vi "RT RFIDs.vi"(8 "error in (no error)":errorcluster, 10 "info":cluster{"File path":T3, "Cfg ":T4} {"Cfg"."Offset_rueda WS 2" format="%.27g"; "Cfg"."Offset_rueda WS 1" format="%.27g"; "Cfg"."Frecuencia de muestreo y módulo CRIO" items=["51.200 kS/s (NI 9234)"=1, "25.600 kS/s (NI 9234)"=2, "17.067 kS/s (NI 9234)"=3, "12.800 kS/s (NI 9234)"=4, "10.240 kS/s (NI 9234)"=5, "8.533 kS/s (NI 9234)"=6, "7.314 kS/s (NI 9234)"=7, "6.400 kS/s (NI 9234)"=8, "5.689 kS/s (NI 9234)"=9, "5.120 kS/s (NI 9234)"=10, "4.654 kS/s (NI 9234)"=11, "4.267 kS/s (NI 9234)"=12, "3.938 kS/s (NI 9234)"=13, "3.657 kS/s (NI 9234)"=14, "3.413 kS/s (NI 9234)"=15, "3.200 kS/s (NI 9234)"=16, "3.012 kS/s (NI 9234)"=17, "2.845 kS/s (NI 9234)"=18, "2.695 kS/s (NI 9234)"=19, "2.560 kS/s (NI 9234)"=20, "2.438 kS/s (NI 9234)"=21, "2.328 kS/s (NI 9234)"=22, "2.226 kS/s (NI 9234)"=23, "2.133 kS/s (NI 9234)"=24, "2.048 kS/s (NI 9234)"=25, "1.969 kS/s (NI 9234)"=26, "1.896 kS/s (NI 9234)"=27, "1.829 kS/s (NI 9234)"=28, "1.765 kS/s (NI 9234)"=29, "1.707 kS/s (NI 9234)"=30, "1.652 kS/s (NI 9234)"=31]}, 11 "Message Queues in":T6) -> (0 "error out":errorcluster)   [LabVIEW 2015]
uses:
  support/Message Queue/All Message Queues.ctl
  support/Message Queue/Message Cluster.ctl
  controls/File paths.ctl
  controls/Cfg_parameters.ctl
  <vilib>/LabVIEW Targets/FPGA/cRIO/shared/nicrio_ModuleControls/nicrio_cRIO-9234_DataRatesRing2.ctl
  controls/RFID State.ctl
  controls/Tags.ctl
  <vilib>/Utility/file.llb/Write Delimited Spreadsheet (string).vi
  support/Message Queue/Enqueue Message (Single).vi
  <vilib>/Utility/error.llb/Error Cluster From Error Code.vi
  <vilib>/ErrorRing/Error Ring.xnode
  support/Message Queue/Message Queue.lvlib
panel:
  in  "TAGs":T1
  in  "RFID State":T2
  out "RFID_LR6_Error":errorcluster
  out "RFID_Error":errorcluster
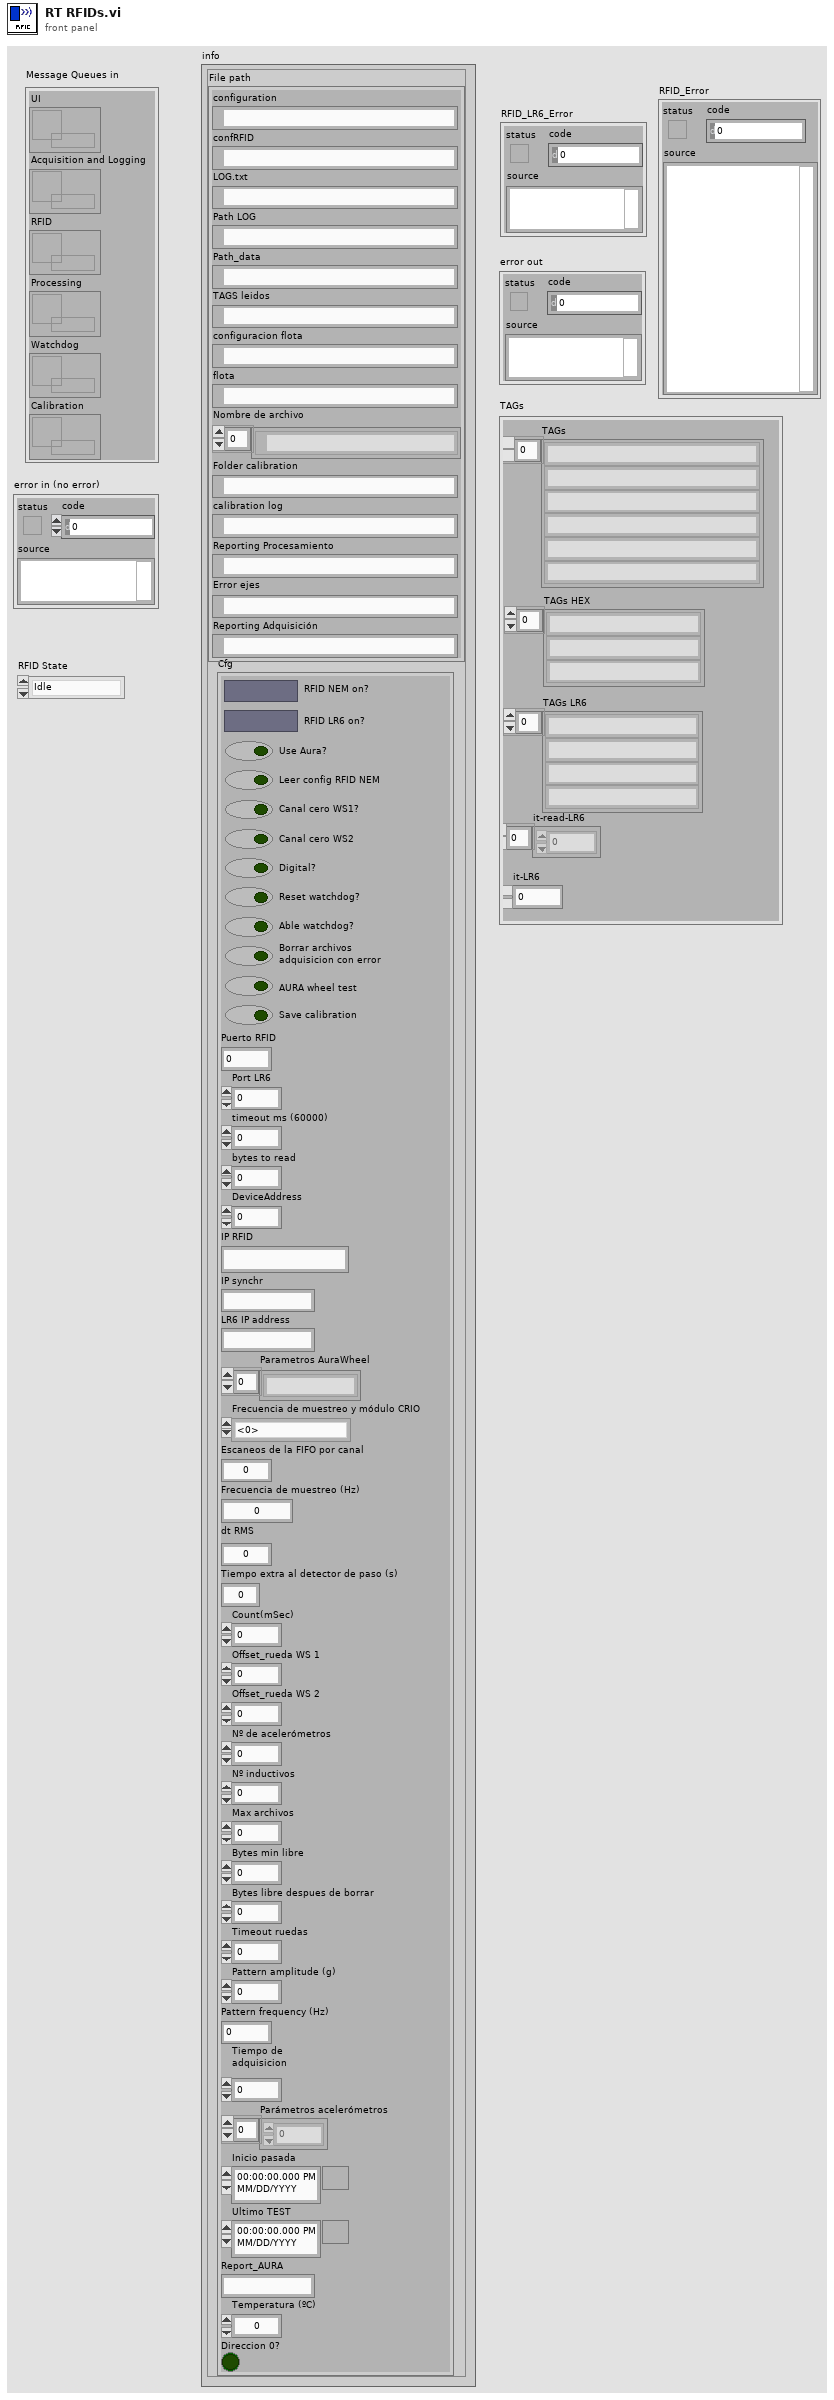
[diagram p1: front panel]
types:
  T1 = typedef "Tags.ctl" = cluster{"TAGs":string[], "TAGs HEX":string[], "TAGs LR6":string[], "it-read-LR6":i32[], "it-LR6":i32}
  T2 = typedef "RFID State.ctl" = enum16{"Idle", "Acquiring"}
  T3 = typedef "File paths.ctl" = cluster{"configuration":path, "confRFID":path, "LOG.txt":path, "Path LOG":path, "Path_data":path, "TAGS leidos":path, "configuracion flota":path, "flota":path, "Nombre de archivo":path[], "Folder calibration":path, "calibration log":path, "Reporting Procesamiento":path, "Error ejes":path, "Reporting Adquisición":path}
  T4 = typedef "Cfg_parameters.ctl" = cluster{"RFID NEM on?":bool, "RFID LR6 on?":bool, "Use Aura?":bool, "Leer config RFID NEM":bool, "Canal cero WS1?":bool, "Canal cero WS2 ":bool, "Digital?":bool, "Reset watchdog?":bool, "Able watchdog?":bool, "Borrar archivos\nadquisicion con error":bool, "AURA wheel test":bool, "Save calibration":bool, "Puerto RFID":u16, "Port LR6":u16, "timeout ms (60000)":i32, "bytes to read":i32, "DeviceAddress":u8, "IP RFID":string, "IP synchr":string, "LR6 IP address":string, "Parametros AuraWheel":string[], "Frecuencia de muestreo y módulo CRIO":T5, "Escaneos de la FIFO por canal":u32, "Frecuencia de muestreo (Hz)":dbl, "dt RMS":dbl, "Tiempo extra al detector de paso (s)":dbl, "Count(mSec)":u32, "Offset_rueda WS 1":fxp<+/-,24,-4>, "Offset_rueda WS 2":fxp<+/-,24,-4>, "Nº de acelerómetros":i32, "Nº inductivos":i32, "Max archivos":u32, "Bytes min libre":u32, "Bytes libre despues de borrar":u32, "Timeout ruedas":dbl, "Pattern amplitude (g)":dbl, "Pattern frequency (Hz)":dbl, "Tiempo de adquisicion\n":dbl, "Parámetros acelerómetros":dbl[], "Inicio pasada":timestamp, "Ultimo TEST":timestamp, "Report_AURA":string, "Temperatura (ºC)":dbl, "Direccion 0?":bool}
  T5 = typedef "nicrio_cRIO-9234_DataRatesRing2.ctl" = u8
  T6 = typedef "Message Queue.lvlib/All Message Queues.ctl" = cluster{"UI":refnum<queue>, "Acquisition and Logging":refnum<queue>, "RFID":refnum<queue>, "Processing":refnum<queue>, "Watchdog":refnum<queue>, "Calibration":refnum<queue>}
  T7 = enum16{"Standard", "Buffered", "CRLF", "Immediate"}
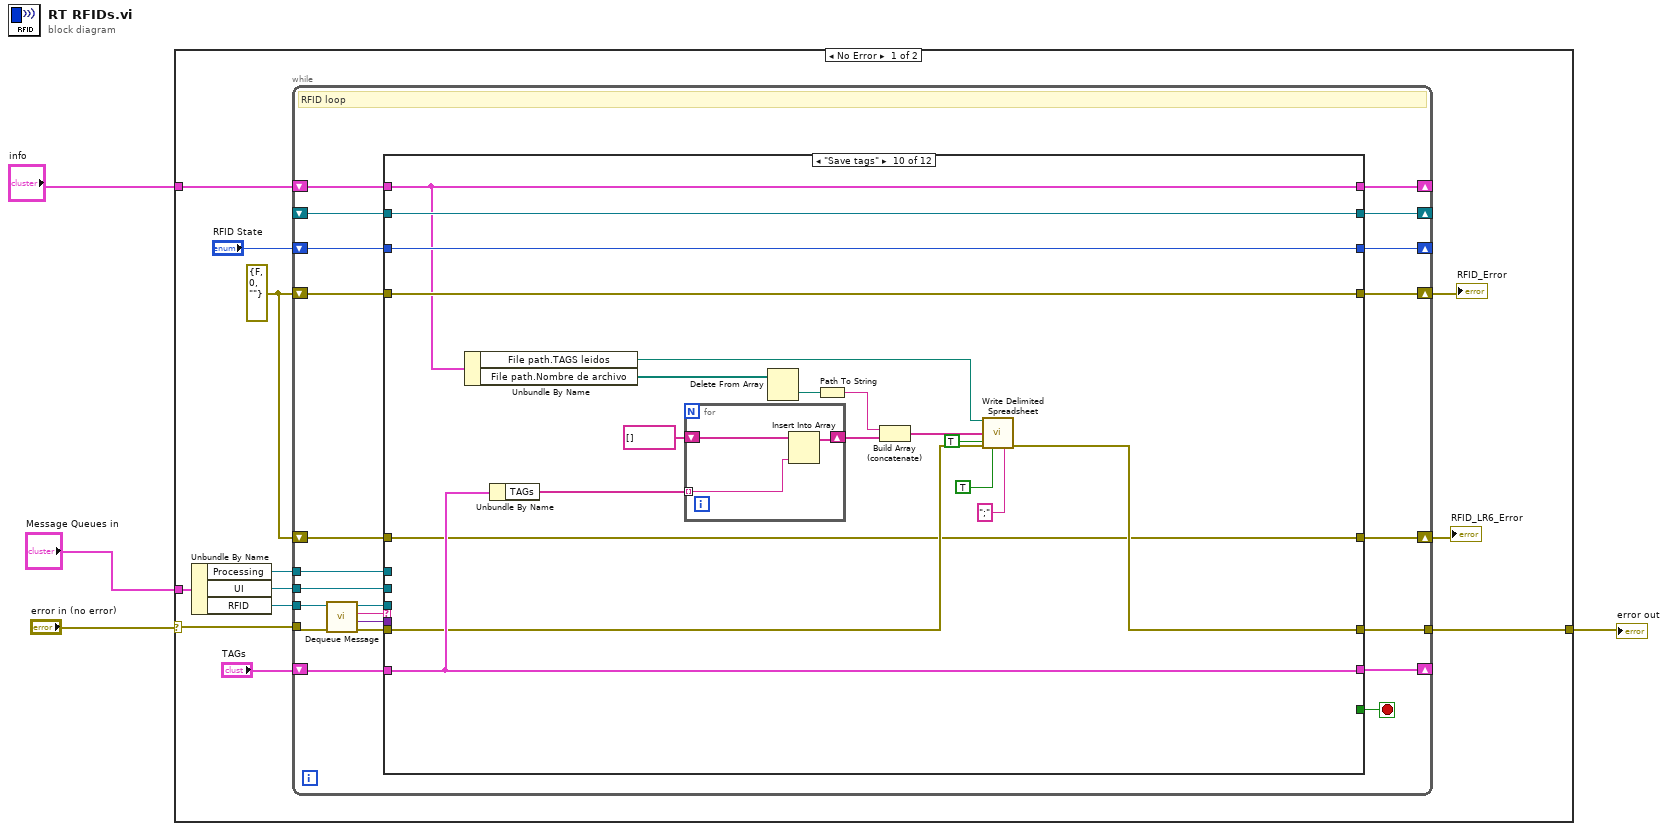
[diagram p0: block diagram]
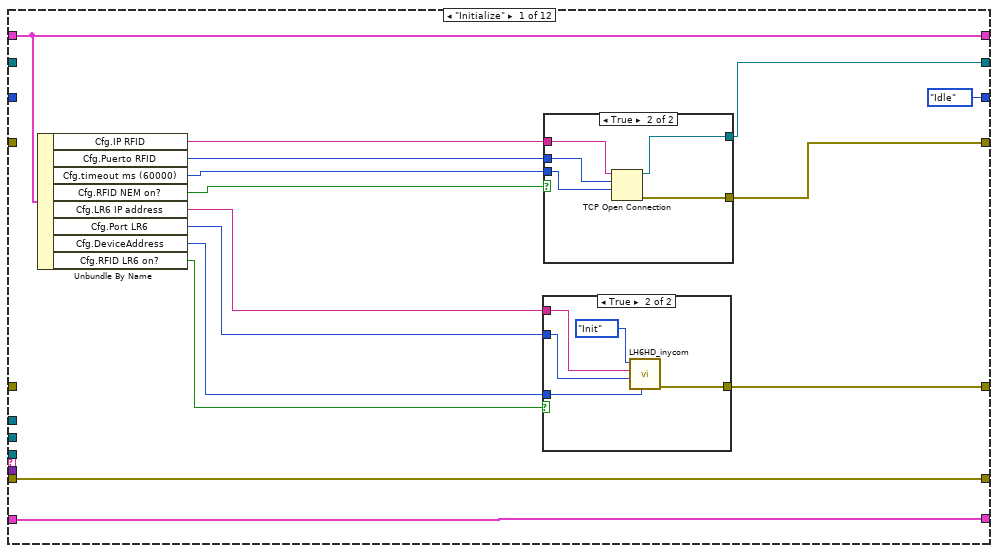
[diagram p2: hidden frame]
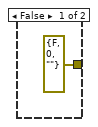
[diagram p3: hidden frame]
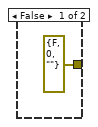
[diagram p4: hidden frame]
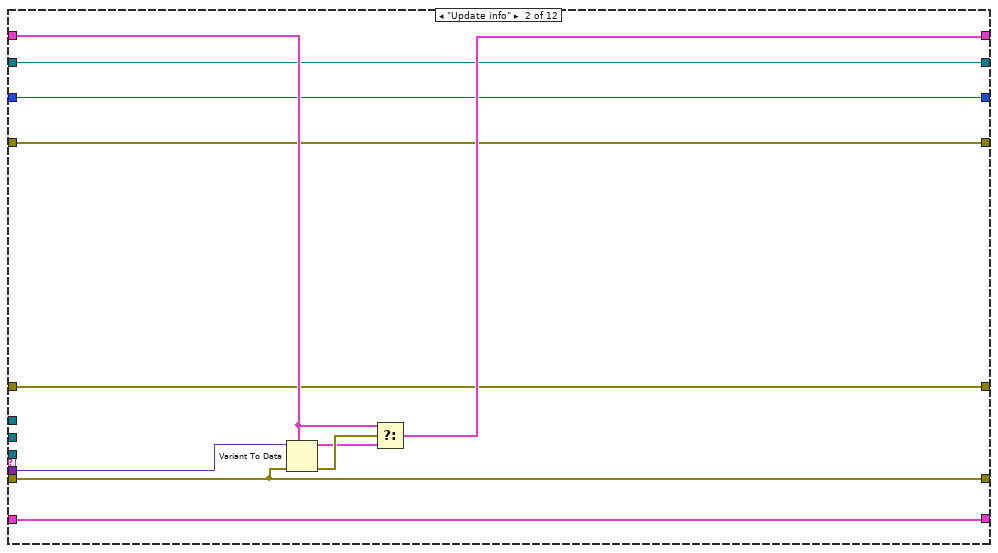
[diagram p5: hidden frame]
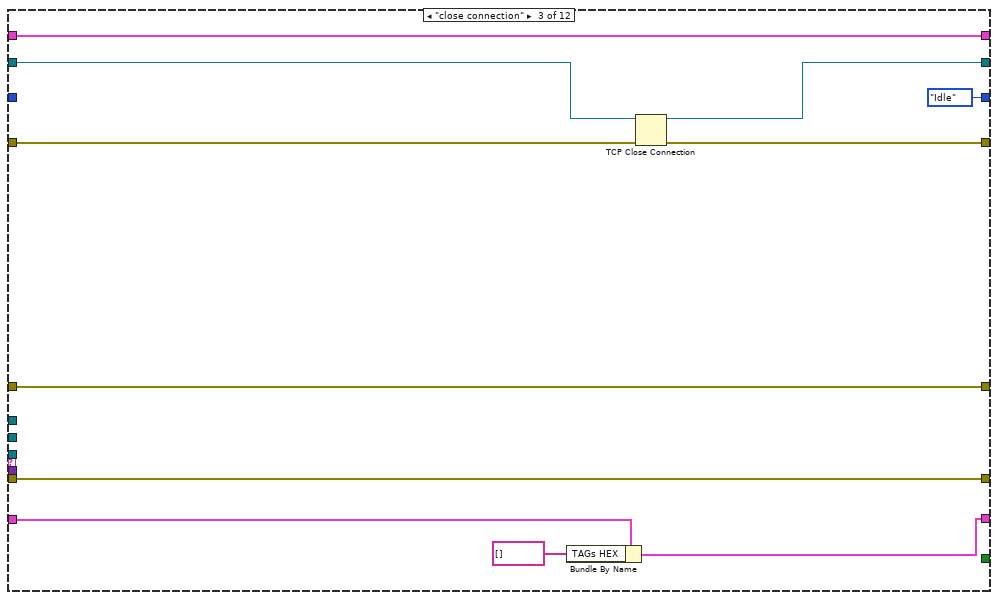
[diagram p6: hidden frame]
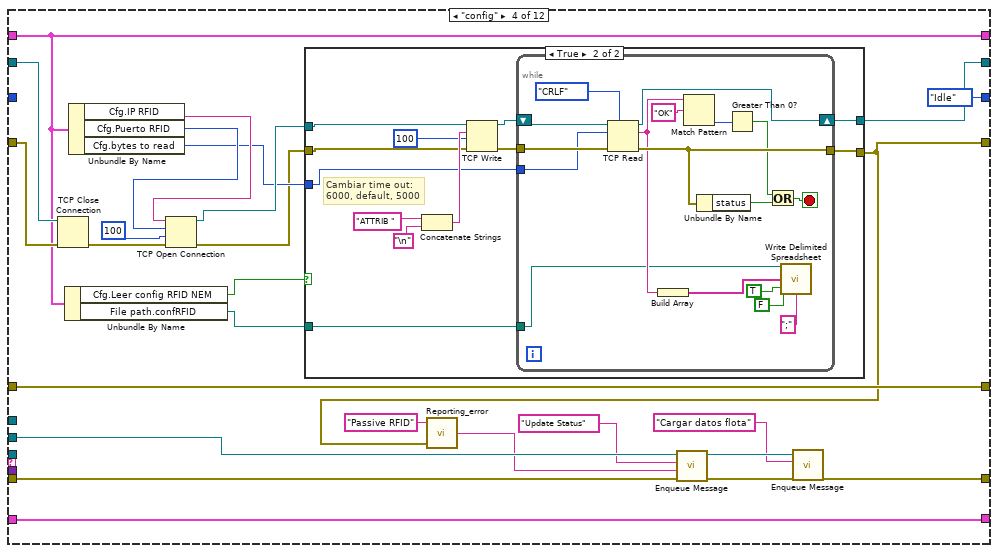
[diagram p7: hidden frame]
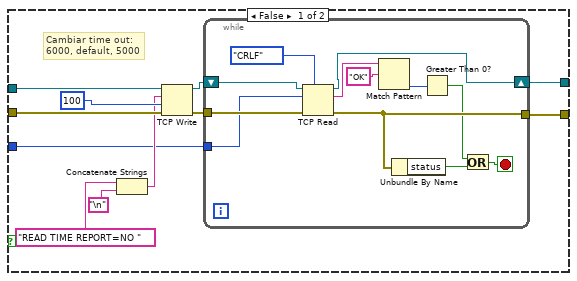
[diagram p8: hidden frame]
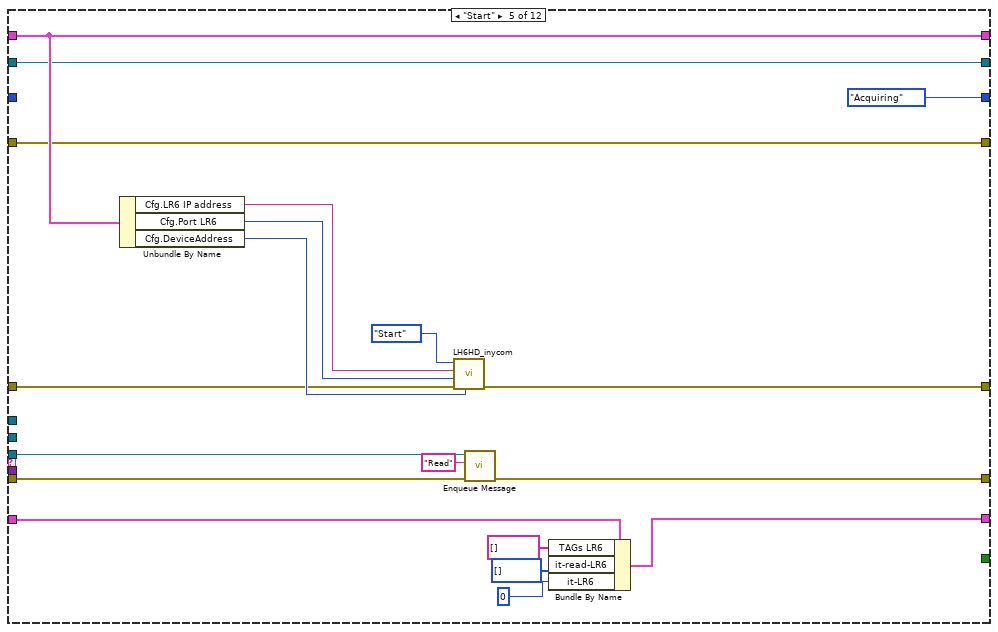
[diagram p9: hidden frame]
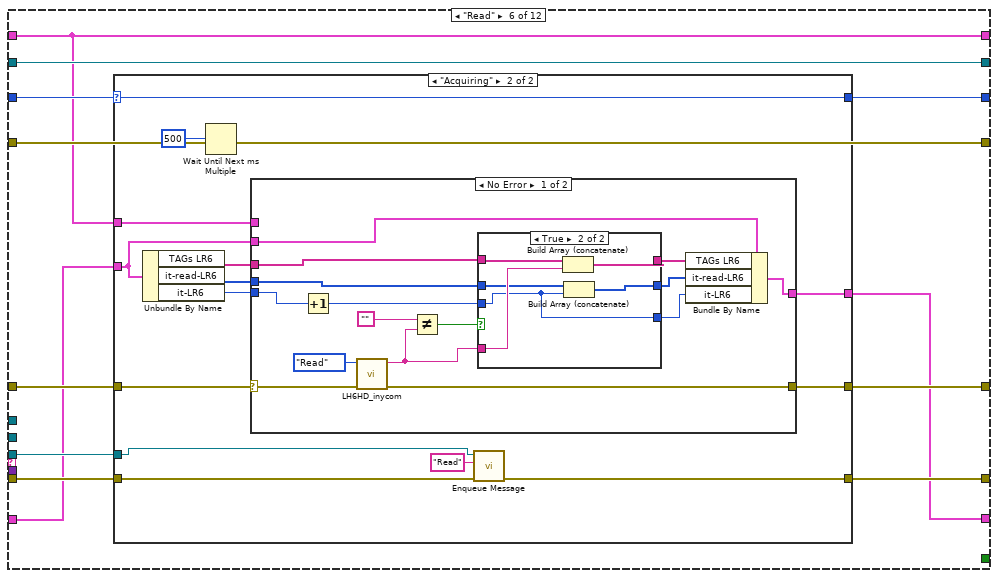
[diagram p10: hidden frame]
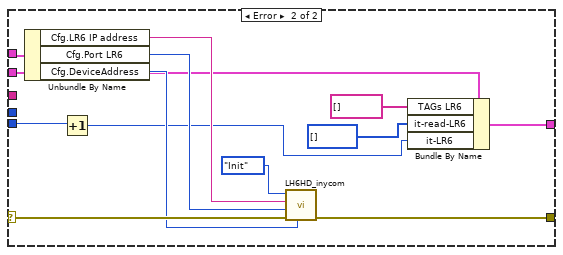
[diagram p13: hidden frame]
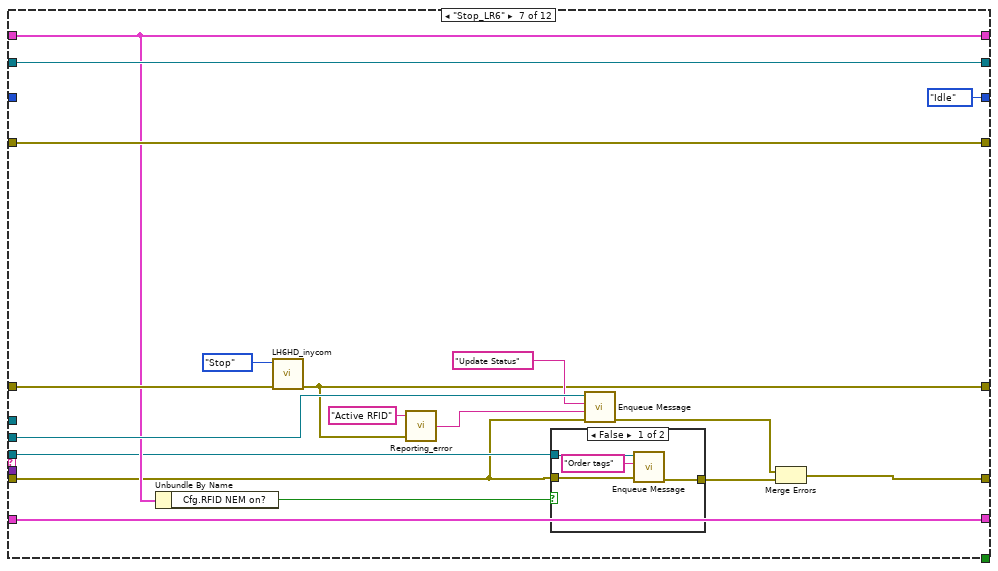
[diagram p14: hidden frame]
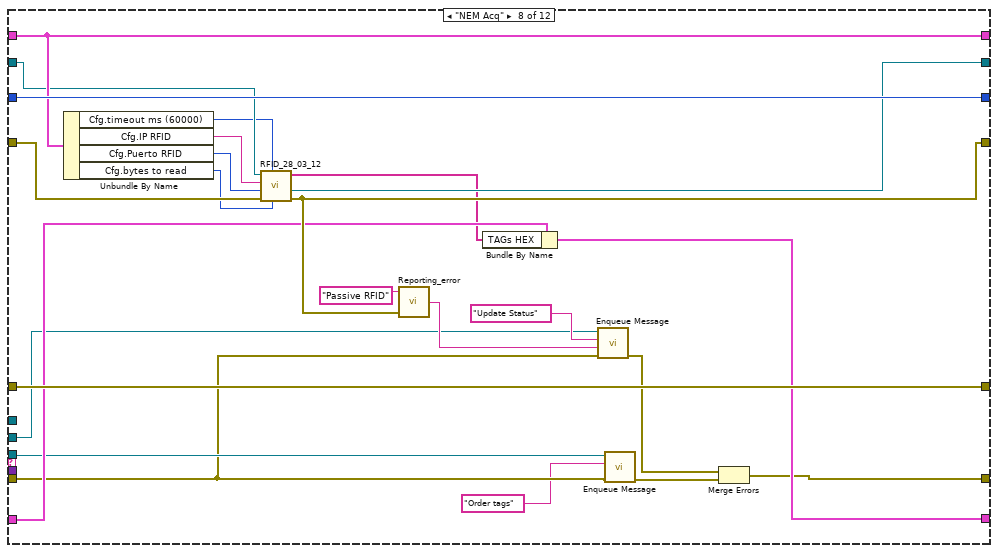
[diagram p16: hidden frame]
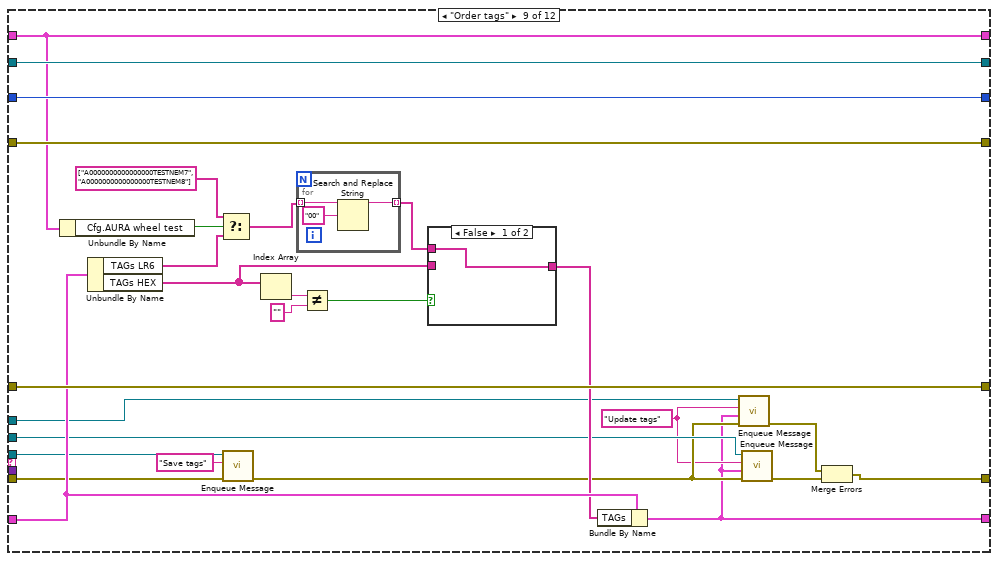
[diagram p17: hidden frame]
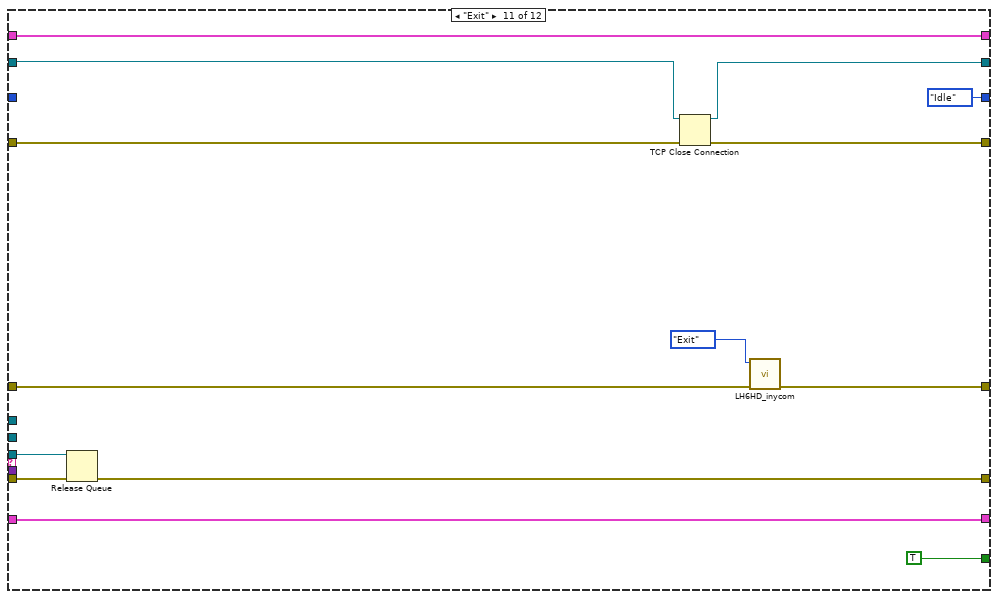
[diagram p19: hidden frame]
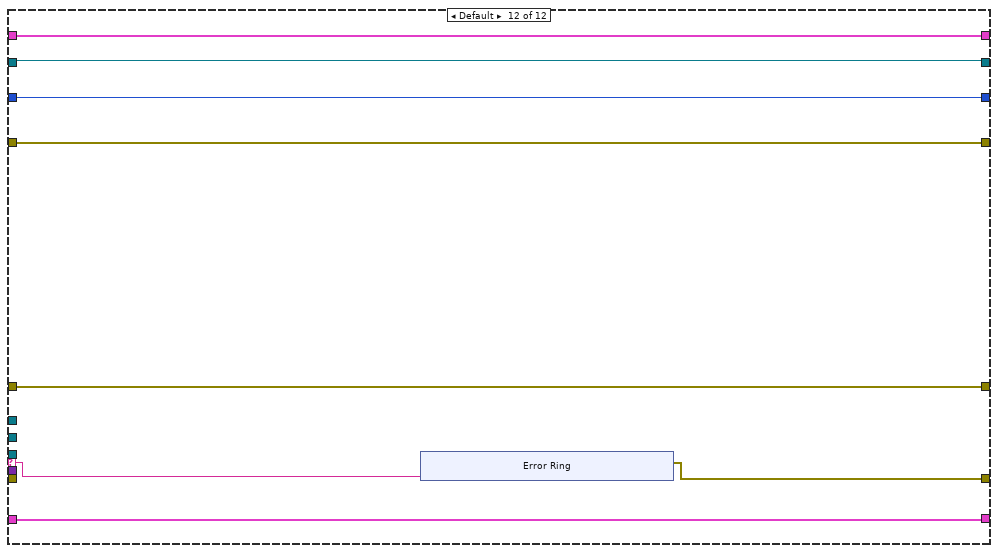
[diagram p20: hidden frame]
diagram:
  n1 = case shown="No Error" "error in (no error)" {
    selector: "error in (no error)" -> [w15 w382]
    tunnel: "Message Queues in" -> [w16 _]
    tunnel: "info" -> [w12 _]
    tunnel: [w11 w382] -> w1
    frame No Error {
      w8 = errorcluster {"status"=FALSE, "code"=0, "source"=""} ("error out")
      n2 = Unbundle By Name(w16) -> ("Processing"=w5:refnum<queue>, "UI"=w13:refnum<queue>, "RFID"=w14:refnum<queue>)
      n3 = while {
        tunnel: w15 -> [w38]
        tunnel: w14 -> [w37]
        tunnel: w13 -> [w35]
        shift-right: [w31] -> _
        shift-left: w12 -> [w32]
        tunnel: [w29] -> w11
        shift-right: [w28] -> _
        shift-left: _ -> [w27]
        shift-right: [w25] -> w9
        shift-left: w8 -> [w24]
        shift-right: [w26] -> w10
        shift-left: w8 -> [w23]
        shift-right: [w21] -> _
        shift-left: "RFID State" -> [w22]
        shift-right: [w19] -> _
        shift-left: "TAGs" -> [w20]
        tunnel: w5 -> [w17]
        stop <- w30 stop-if-true
        # "RFID loop"
        n4 = call "Dequeue Message.vi"("error in (no error)"=w38, "Message Queue"=w37) -> ("error out"=w34:errorcluster, "Message Data"=w18:variant, "Message"=w33:string, "dup Message Queue"=w36:refnum<queue>)  [unwired: 6 in]
        n5 = case shown="\"Save tags\"" w33 {
          selector: w33 -> [_ _ _ _ _ _ _ _ _ _ _ w372]
          tunnel: w36 -> [_ _ _ _ w174 w188 w257 w280 w305 _ w364 _]
          tunnel: w35 -> [_ _ _ w94 _ _ w262 w281 w308 _ _ _]
          tunnel: w34 -> [w53 w73 w83 w91 w176 w190 w256 w276 w307 w333 w365 _]
          tunnel: [w53 w73 w83 w90 w175 w189 w253 w279 w299 w332 w363 w373] -> w29
          tunnel: w32 -> [w52 w70 w87 w102 w180 w187 w258 w295 w321 w336 w366 w374]
          tunnel: [w52 w71 w87 w102 w180 w187 w258 w295 w321 w336 w366 w374] -> w31
          tunnel: [_ _ _ _ _ _ _ _ _ _ TRUE _] -> w30
          tunnel: [w47 w67 w86 w98 w178 w193 w267 w293 w323 w347 w361 w370] -> w25
          tunnel: [w46 w68 w85 w103 w177 w194 w268 w292 w325 w349 w360 w371] -> w28
          tunnel: w27 -> [_ w68 w84 w110 w177 w194 w268 w291 w325 w349 w359 w371]
          tunnel: [w41 w66 w81 w113 w181 w191 w260 w297 w322 w331 w357 w369] -> w26
          tunnel: w24 -> [_ w67 w82 w105 w178 w193 w267 w294 w323 w347 w356 w370]
          tunnel: w23 -> [_ w66 w81 w113 w179 w192 w265 w297 w322 w331 w355 w369]
          tunnel: w22 -> [_ w69 _ _ _ w196 _ w298 w324 w348 _ w368]
          tunnel: [RFID_State."Idle" ("RFID State") w69 RFID_State."Idle" ("RFID State") RFID_State."Idle" ("RFID State") RFID_State."Acquiring" ("RFID State") w195 RFID_State."Idle" ("RFID State") w298 w324 w348 RFID_State."Idle" ("RFID State") w368] -> w21
          tunnel: w20 -> [w39 w72 w79 w88 w172 w186 w263 w284 w311 w338 w353 w367]
          tunnel: [w39 w72 w78 w88 w171 w185 w263 w282 w302 w338 w353 w367] -> w19
          tunnel: w18 -> [_ w74 _ _ _ _ _ _ _ _ _ _]
          tunnel: w17 -> [_ _ _ _ _ _ _ _ w309 _ _ _]
          frame "Initialize" {
            n6 = Unbundle By Name(w52) -> ("Cfg.IP RFID"=w51:string, "Cfg.Puerto RFID"=w49:u16, "Cfg.timeout ms (60000)"=w48:i32, "Cfg.RFID NEM on?"=w50:bool, "Cfg.LR6 IP address"=w44:string, "Cfg.Port LR6"=w43:u16, "Cfg.DeviceAddress"=w42:u8, "Cfg.RFID LR6 on?"=w45:bool)
            n7 = case shown="True" w45 {
              tunnel: w44 -> [_ w58]
              tunnel: w43 -> [_ w56]
              tunnel: w42 -> [_ w57]
              tunnel: [errorcluster {"status"=FALSE, "code"=0, "source"=""} ("error out") w55] -> w41
              frame False {
              }
              frame True {
                n8 = call "LH6HD_inycom.vi"("DeviceAddress"=w57, "Reader Port"=w56, "IP Address"=w58, "Action"=enum16{"Init", "Start", "Read", "Stop", "Exit"}."Init") -> ("error out"=w55:errorcluster)  [unwired: 6 in, 1 out]
              }
            }
            n9 = case shown="True" w50 {
              tunnel: w51 -> [_ w65]
              tunnel: w49 -> [_ w64]
              tunnel: w48 -> [_ w63]
              tunnel: [errorcluster {"status"=FALSE, "code"=0, "source"=""} ("error out") w62] -> w47
              tunnel: [_ w61] -> w46
              frame False {
              }
              frame True {
                n10 = TCP Open Connection(address=w65, remote port or service name=w64, timeout ms (60000)=w63) -> (connection ID=w61:refnum<k5>, error out=w62:errorcluster)  [unwired: 1 in, 1 out]
              }
            }
          }
          frame "Update info" {
            n11 = Variant To Data(error in=w73, type=w70, Variant=w74) -> (data=w75:cluster{"File path":T3, "Cfg ":T4}, error out=w76:errorcluster)
            n12 = Select(t=w70, s=w76, f=w75) -> (s? t:f=w71:cluster{"File path":T3, "Cfg ":T4})
          }
          frame "close connection" {
            n13 = Bundle By Name(cluster=w79, "TAGs HEX"=string[] [] ("TAGs")) -> (w78:T1)
            n14 = TCP Close Connection(connection ID=w84, error in (no error)=w82) -> (connection ID out=w85:refnum<k5>, error out=w86:errorcluster)  [unwired: 1 out]
          }
          frame "config" {
            n15 = TCP Close Connection(connection ID=w110, error in (no error)=w105) -> (error out=w112:errorcluster)  [unwired: 1 in, 1 out]
            n16 = Unbundle By Name(w102) -> ("Cfg.Leer config RFID NEM"=w101:bool, "File path.confRFID"=w100:path)
            n17 = Unbundle By Name(w102) -> ("Cfg.IP RFID"=w109:string, "Cfg.Puerto RFID"=w108:u16, "Cfg.bytes to read"=w106:i32)
            n18 = TCP Open Connection(address=w109, remote port or service name=w108, timeout ms (60000)=100, error in (no error)=w112) -> (connection ID=w107:refnum<k5>, error out=w104:errorcluster)  [unwired: 1 out]
            n19 = case shown="True" w101 {
              tunnel: w107 -> [w124 w142]
              tunnel: [w122 w140] -> w98
              tunnel: w104 -> [w119 w141]
              tunnel: [w115 w139] -> w103
              tunnel: w106 -> [w114 w137]
              tunnel: w100 -> [_ w138]
              frame False {
                # "Cambiar time out:\n6000, default, 5000"
                n20 = Concatenate Strings("READ TIME REPORT=NO " ("data in"), "\n") -> (w116:string)
                n21 = TCP Write(connection ID=w124, data in=w116, error in (no error)=w119, 9:100 ("timeout ms (25000)")) -> (connection ID out=w120:refnum<k5>, error out=w121:errorcluster)  [unwired: 1 out]
                n22 = while {
                  tunnel: w121 -> [w135]
                  tunnel: [w133] -> w122
                  shift-right: [w126] -> w115
                  shift-left: w120 -> [w134]
                  tunnel: w114 -> [w125]
                  stop <- w130 stop-if-true
                  n23 = TCP Read(connection ID=w134, bytes to read=w125, error in (no error)=w135, 7:T7."CRLF" ("mode (standard)")) -> (connection ID out=w126:refnum<k5>, data out=w128:string, error out=w133:errorcluster)  [unwired: 1 in]
                  n24 = Match Pattern(string=w128, regular expression="OK") -> (offset past match=w131:i32)  [unwired: 4 out]
                  n25 = Unbundle By Name(w133) -> ("status"=w129:bool)
                  n26 = Greater Than 0?(x=w131) -> (x > 0?=w127:bool)
                  n27 = Or(x=w127, y=w129) -> (x .or. y?=w130:bool)
                }
              }
              frame True {
                # "Cambiar time out:\n6000, default, 5000"
                n28 = Concatenate Strings("ATTRIB " ("data in"), "\n") -> (w148:string)
                n29 = TCP Write(connection ID=w142, data in=w148, error in (no error)=w141, 9:100 ("timeout ms (25000)")) -> (connection ID out=w145:refnum<k5>, error out=w144:errorcluster)  [unwired: 1 out]
                n30 = while {
                  tunnel: w144 -> [w164]
                  tunnel: [w162] -> w140
                  shift-right: [w151] -> w139
                  shift-left: w145 -> [w163]
                  tunnel: w138 -> [w150]
                  tunnel: w137 -> [w149]
                  stop <- w159 stop-if-true
                  n31 = TCP Read(connection ID=w163, bytes to read=w149, error in (no error)=w164, 7:T7."CRLF" ("mode (standard)")) -> (connection ID out=w151:refnum<k5>, data out=w153:string, error out=w162:errorcluster)  [unwired: 1 in]
                  n32 = Build Array(w153) -> (w152:string[])
                  n33 = Match Pattern(string=w153, regular expression="OK") -> (offset past match=w160:i32)  [unwired: 4 out]
                  n34 = Unbundle By Name(w162) -> ("status"=w158:bool)
                  n35 = Greater Than 0?(x=w160) -> (x > 0?=w157:bool)
                  n36 = Or(x=w157, y=w158) -> (x .or. y?=w159:bool)
                  n37 = call-poly <vilib>:"Write Delimited Spreadsheet.vi"("file path (dialog if empty)"=w150, "1D data"=w152, "append to file? (F)"=FALSE ("transpose? (no:F)"), "transpose? (F)"=TRUE ("append to file? (new file:F)"), "delimiter (\\t)"=";" ("delimiter (\\t)")) -> ()  [unwired: 9 in, 2 out]
                }
              }
            }
            n38 = call "Reporting_error.vi"("error out 2"=w98, "Concept"="Passive RFID") -> ("Reporting"=w92:string)  [unwired: 1 in]
            n39 = call-poly "Enqueue Message.vi"("error in (no error)"=w91, "Message Data"=w92, "Message"="Update Status", "Message Queue"=w94) -> ("error out"=w97:errorcluster, "dup Message Queue"=w96:refnum<queue>)  [unwired: 6 in]
            n40 = call-poly "Enqueue Message.vi"("error in (no error)"=w97, "Message"="Cargar datos flota", "Message Queue"=w96) -> ("error out"=w90:errorcluster)  [unwired: 7 in, 1 out]
          }
          frame "Start" {
            n41 = Unbundle By Name(w180) -> ("Cfg.LR6 IP address"=w184:string, "Cfg.Port LR6"=w183:u16, "Cfg.DeviceAddress"=w182:u8)
            n42 = call "LH6HD_inycom.vi"("DeviceAddress"=w182, "error in (no error)"=w179, "Reader Port"=w183, "IP Address"=w184, "Action"=enum16{"Init", "Start", "Read", "Stop", "Exit"}."Start") -> ("error out"=w181:errorcluster)  [unwired: 5 in, 1 out]
            n43 = call-poly "Enqueue Message.vi"("error in (no error)"=w176, "Message"="Read", "Message Queue"=w174) -> ("error out"=w175:errorcluster)  [unwired: 7 in, 1 out]
            n44 = Bundle By Name(cluster=w172, "TAGs LR6"=string[] [], "it-read-LR6"=i32[] [], "it-LR6"=0) -> (w171:T1)
          }
          frame "Read" {
            n45 = case shown="\"Acquiring\"" w196 {
              selector: w196 -> [w199 w214]
              tunnel: [w199 w214] -> w195
              tunnel: w192 -> [w200 w208]
              tunnel: [w200 w207] -> w191
              tunnel: w190 -> [w198 w212]
              tunnel: [w198 w211] -> w189
              tunnel: w188 -> [_ w210]
              tunnel: w187 -> [_ w206]
              tunnel: w186 -> [w197 w205]
              tunnel: [w197 w204] -> w185
              frame "Idle", Default {
              }
              frame "Acquiring" {
                n46 = Unbundle By Name(w205) -> ("TAGs LR6"=w203:string[], "it-read-LR6"=w202:i32[], "it-LR6"=w201:i32)
                n47 = Wait Until Next ms Multiple(millisecond multiple=u32 500) -> ()  [unwired: 1 out]
                n48 = case shown="No Error" w208 {
                  selector: w208 -> [w228 w250]
                  tunnel: [w227 w248] -> w207
                  tunnel: w206 -> [_ w249]
                  tunnel: w205 -> [w223 w244]
                  tunnel: [w222 w243] -> w204
                  tunnel: w203 -> [w219 _]
                  tunnel: w202 -> [w218 _]
                  tunnel: w201 -> [w217 w240]
                  frame No Error {
                    n49 = Increment(x=w217) -> (x+1=w216:i32)
                    n50 = call "LH6HD_inycom.vi"("error in (no error)"=w228, "Action"=enum16{"Init", "Start", "Read", "Stop", "Exit"}."Read") -> ("error out"=w227:errorcluster, "Tag"=w224:string)  [unwired: 8 in]
                    n51 = Not Equal?(x="", y=w224) -> (x != y?=w225:bool)
                    n52 = case shown="True" w225 {
                      tunnel: [w232 w238] -> w221
                      tunnel: w219 -> [w232 w234]
                      tunnel: w218 -> [w231 w235]
                      tunnel: [w231 w237] -> w220
                      tunnel: w224 -> [_ w236]
                      tunnel: w216 -> [w230 w233]
                      tunnel: [w230 w233] -> w215
                      frame False {
                      }
                      frame True {
                        n53 = Build Array (concatenate)(w234, w236) -> (w238:string[])
                        n54 = Build Array (concatenate)(w235, w233) -> (w237:i32[])
                      }
                    }
                    n55 = Bundle By Name(cluster=w223, "TAGs LR6"=w221, "it-read-LR6"=w220, "it-LR6"=w215) -> (w222:T1)
                  }
                  frame Error {
                    n56 = Unbundle By Name(w249) -> ("Cfg.LR6 IP address"=w246:string, "Cfg.Port LR6"=w245:u16, "Cfg.DeviceAddress"=w247:u8)
                    n57 = Increment(x=w240) -> (x+1=w239:i32)
                    n58 = call "LH6HD_inycom.vi"("DeviceAddress"=w247, "error in (no error)"=w250, "Reader Port"=w245, "IP Address"=w246, "Action"=enum16{"Init", "Start", "Read", "Stop", "Exit"}."Init") -> ("error out"=w248:errorcluster)  [unwired: 5 in, 1 out]
                    n59 = Bundle By Name(cluster=w244, "TAGs LR6"=string[] [], "it-read-LR6"=i32[] [], "it-LR6"=w239) -> (w243:T1)
                  }
                }
                n60 = call-poly "Enqueue Message.vi"("error in (no error)"=w212, "Message"="Read", "Message Queue"=w210) -> ("error out"=w211:errorcluster)  [unwired: 7 in, 1 out]
              }
            }
          }
          frame "Stop_LR6" {
            n61 = Unbundle By Name(w258) -> ("Cfg.RFID NEM on?"=w252:bool)
            n62 = call "LH6HD_inycom.vi"("error in (no error)"=w265, "Action"=enum16{"Init", "Start", "Read", "Stop", "Exit"}."Stop") -> ("error out"=w260:errorcluster)  [unwired: 8 in, 1 out]
            n63 = call "Reporting_error.vi"("error out 2"=w260, "Concept"="Active RFID") -> ("Reporting"=w259:string)  [unwired: 1 in]
            n64 = case shown="False" w252 {
              tunnel: w257 -> [w273 _]
              tunnel: w256 -> [w272 w274]
              tunnel: [w271 w274] -> w254
              frame False {
                n65 = call-poly "Enqueue Message.vi"("error in (no error)"=w272, "Message"="Order tags", "Message Queue"=w273) -> ("error out"=w271:errorcluster)  [unwired: 7 in, 1 out]
              }
              frame True {
              }
            }
            n66 = call-poly "Enqueue Message.vi"("error in (no error)"=w256, "Message Data"=w259, "Message"="Update Status", "Message Queue"=w262) -> ("error out"=w255:errorcluster)  [unwired: 6 in, 1 out]
            n67 = Merge Errors(w255, w254) -> (w253:errorcluster)
          }
          frame "NEM Acq" {
            n68 = Unbundle By Name(w295) -> ("Cfg.timeout ms (60000)"=w290:i32, "Cfg.IP RFID"=w289:string, "Cfg.Puerto RFID"=w288:u16, "Cfg.bytes to read"=w287:i32)
            n69 = call "RFID_28_03_12.vi"("BYTES TO READ"=w287, "TIMEOUT"=w290, "RFID_Error"=w294, "Puerto RFID"=w288, "IP RFID"=w289, "RFID ID"=w291) -> ("RFID Error"=w293:errorcluster, "connection ID out"=w292:refnum<k5>, "TAGs HEX"=w283:string[])  [unwired: 1 in, 1 out]
            n70 = call "Reporting_error.vi"("error out 2"=w293, "Concept"="Passive RFID") -> ("Reporting"=w285:string)  [unwired: 1 in]
            n71 = Bundle By Name(cluster=w284, "TAGs HEX"=w283) -> (w282:T1)
            n72 = call-poly "Enqueue Message.vi"("error in (no error)"=w276, "Message Data"=w285, "Message"="Update Status", "Message Queue"=w281) -> ("error out"=w278:errorcluster)  [unwired: 6 in, 1 out]
            n73 = call-poly "Enqueue Message.vi"("error in (no error)"=w276, "Message"="Order tags", "Message Queue"=w280) -> ("error out"=w277:errorcluster)  [unwired: 7 in, 1 out]
            n74 = Merge Errors(w278, w277) -> (w279:errorcluster)
          }
          frame "Order tags" {
            w303 = "Update tags" ("Message")
            n75 = Unbundle By Name(w321) -> ("Cfg.AURA wheel test"=w320:bool)
            n76 = Unbundle By Name(w311) -> ("TAGs LR6"=w319:string[], "TAGs HEX"=w312:string[])
            n77 = Select(t=string[] ["A0000000000000000TESTNEM7", "A0000000000000000TESTNEM8"], s=w320, f=w319) -> (s? t:f=w317:string[])
            n78 = call-poly "Enqueue Message.vi"("error in (no error)"=w307, "Message"="Save tags", "Message Queue"=w305) -> ("error out"=w306:errorcluster)  [unwired: 7 in, 1 out]
            n79 = Index Array(array=w312) -> (element=w316:string)  [unwired: 1 in]
            n80 = for {
              tunnel: w317 -> [w330] mode=indexing
              tunnel: [w328] -> w313 mode=indexing
              n81 = Search and Replace String(input string=w330, search string="00") -> (result string=w328:string)  [unwired: 6 in, 3 out]
            }
            n82 = Not Equal?(x=w316, y="" ("delimiter (\\t)")) -> (x != y?=w314:bool)
            n83 = case shown="False" w314 {
              tunnel: w313 -> [w326 _]
              tunnel: [w326 w327] -> w310
              tunnel: w312 -> [_ w327]
              frame False {
              }
              frame True {
              }
            }
            n84 = Bundle By Name(cluster=w311, "TAGs"=w310) -> (w302:T1)
            n85 = call-poly "Enqueue Message.vi"("error in (no error)"=w306, "Message Data"=w302, "Message"=w303, "Message Queue"=w309) -> ("error out"=w300:errorcluster)  [unwired: 6 in, 1 out]
            n86 = call-poly "Enqueue Message.vi"("error in (no error)"=w306, "Message Data"=w302, "Message"=w303, "Message Queue"=w308) -> ("error out"=w301:errorcluster)  [unwired: 6 in, 1 out]
            n87 = Merge Errors(w300, w301) -> (w299:errorcluster)
          }
          frame "Save tags" {
            n88 = Unbundle By Name(w336) -> ("File path.TAGS leidos"=w334:path, "File path.Nombre de archivo"=w335:path[])
            n89 = Unbundle By Name(w338) -> ("TAGs"=w337:string[])
            n90 = for {
              shift-right: [w352] -> w345
              shift-left: string[] [] -> [w351]
              tunnel: w337 -> [w350] mode=indexing
              n91 = Insert Into Array(array=w351, new element=w350) -> (w352:string[])  [unwired: 1 in]
            }
            n92 = Delete From Array(array=w335) -> (deleted portion=w343:path)  [unwired: 2 in, 1 out]
            n93 = Path To String(path=w343) -> (string=w344:string)
            n94 = Build Array (concatenate)(w344, w345) -> (w339:string[])
            n95 = call-poly <vilib>:"Write Delimited Spreadsheet.vi"("file path (dialog if empty)"=w334, "1D data"=w339, "append to file? (F)"=TRUE ("transpose? (no:F)"), "error in (no error)"=w333, "transpose? (F)"=TRUE ("append to file? (new file:F)"), "delimiter (\\t)"=";" ("delimiter (\\t)")) -> ("error out"=w332:errorcluster)  [unwired: 8 in, 1 out]
          }
          frame "Exit" {
            n96 = Release Queue(queue=w364, error in (no error)=w365) -> (error out=w363:errorcluster)  [unwired: 1 in, 2 out]
            n97 = TCP Close Connection(connection ID=w359, error in (no error)=w356) -> (connection ID out=w360:refnum<k5>, error out=w361:errorcluster)  [unwired: 1 out]
            n98 = call "LH6HD_inycom.vi"("error in (no error)"=w355, "Action"=enum16{"Init", "Start", "Read", "Stop", "Exit"}."Exit") -> ("error out"=w357:errorcluster)  [unwired: 8 in, 1 out]
          }
          frame Default {
            n99 = xnode "Error Ring"("parameter 0"=w372) -> ("error out"=w373:errorcluster)
          }
        }
      }
      "RFID_LR6_Error" <- w10
      "RFID_Error" <- w9
    }
    frame Error {
    }
  }
  "error out" <- w1
